vi "KepcoDCPwr Query Voltage Limit.vi"(0 "VISA Session":refnum<visa-resource-name>, 5 "Model In":string, 7 "channel name (\"\")":string="\"\"", 9 "Max Level (T),MIN LEVEL(F)":bool caption="Level", 11 "error in (no error)":errorcluster {"code" format="%.0x"}) -> (4 "VISA Session Out":refnum<visa-resource-name>, 6 "Model Out":string, 8 "channel name out (\"\")":string="\"\"" caption="channel name Out (\"\")", 10 "voltage level":dbl format="%^.2e", 15 "error out":errorcluster {"code" format="%.0x"})   [LabVIEW 2013]
doc: "This VI returns the maximum programmable voltage level that the power supply accepts for a particular current limit on a channel for the output range to which the power supply is currently configured."
uses:
  <vilib>/regexp/Match Regular Expression.xnode
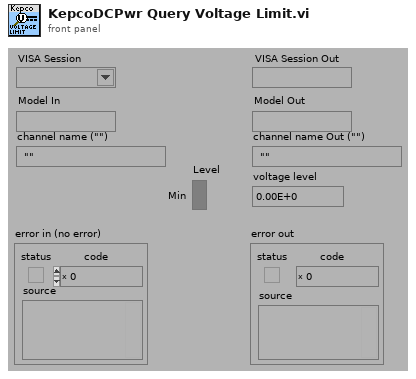
[diagram p1: front panel]
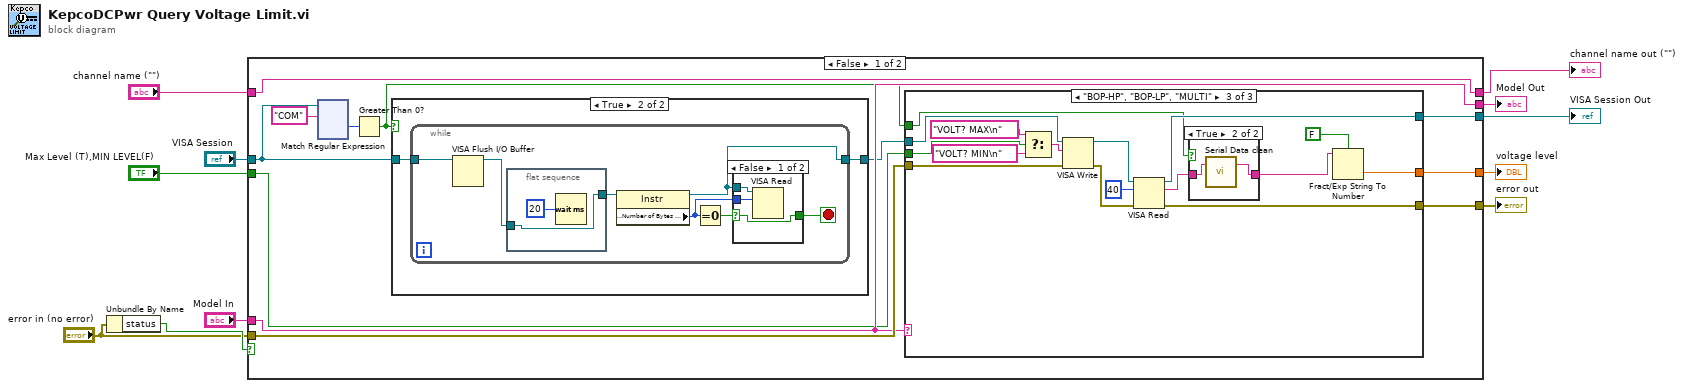
[diagram p0: block diagram]
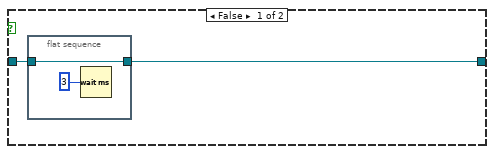
[diagram p2: hidden frame]
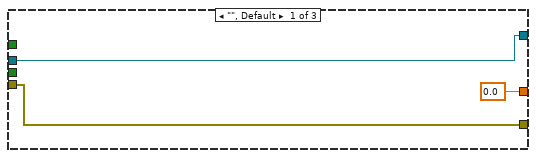
[diagram p4: hidden frame]
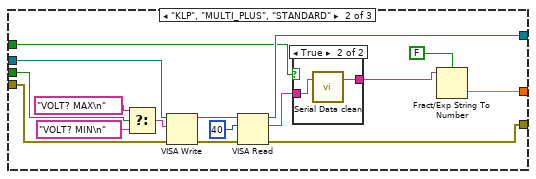
[diagram p5: hidden frame]
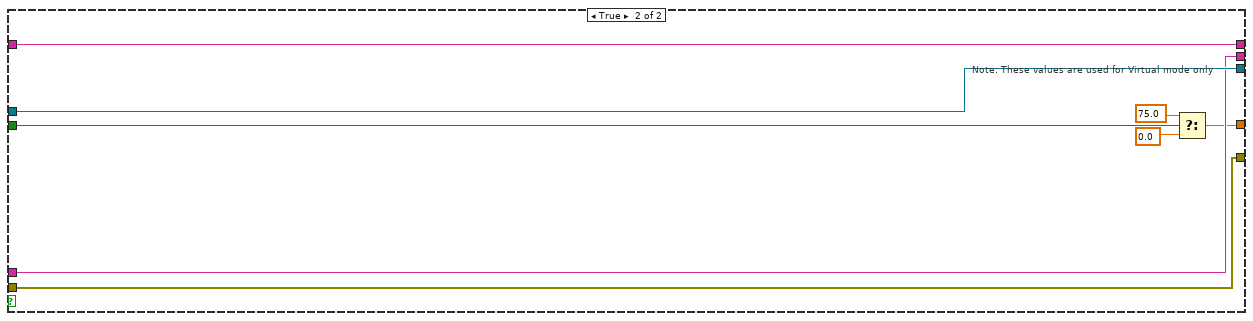
[diagram p8: hidden frame]
diagram:
  n1 = Unbundle By Name("error in (no error)") -> ("status"=w10:bool)
  n2 = case shown="False" w10 {
    tunnel: [w19 w202] -> w11
    tunnel: "error in (no error)" -> [w22 w202]
    tunnel: [w20 w201] -> w5
    tunnel: "VISA Session" -> [w12 w201]
    tunnel: [w21 w200] -> w4
    tunnel: "Model In" -> [w21 w200]
    tunnel: [w23 w199] -> w3
    tunnel: "channel name (\"\")" -> [w23 w199]
    tunnel: [w18 w196] -> w2
    tunnel: "Max Level (T),MIN LEVEL(F)" -> [w17 w198]
    frame False {
      n3 = xnode "Match Regular Expression"("input string"=w12, "regular expression"="COM") -> ("offset past match"=w15:i32)  [unwired: 2 in, 6 out]
      n4 = Greater Than 0?(x=w15) -> (x > 0?=w14:bool)
      n5 = case shown="True" w14 {
        tunnel: [w25 w29] -> w13
        tunnel: w12 -> [w24 w28]
        frame False {
          n6 = flat-sequence {
            tunnel: w24 -> [w27]
            tunnel: [w27] -> w25
            frame #0 {
              n7 = Wait (ms)(milliseconds to wait=u32 3 ("byte count (0)")) -> ()  [unwired: 1 out]
            }
          }
        }
        frame True {
          n8 = while {
            tunnel: w28 -> [w32]
            tunnel: [w34] -> w29
            stop <- w35 stop-if-true
            n9 = VISA Flush I/O Buffer(VISA resource name=w32) -> (VISA resource name out=w31:refnum<visa-resource-name>)  [unwired: 2 in, 1 out]
            n10 = flat-sequence {
              tunnel: w31 -> [w37]
              tunnel: [w37] -> w30
              frame #0 {
                n11 = Wait (ms)(milliseconds to wait=u32 20) -> ()  [unwired: 1 out]
              }
            }
            n12 = property class="Instr"(reference=w30) -> (reference out=w34:refnum<visa-resource-name>, "Serial Settings:Number of Bytes at Serial Port"=w33:u32)  [unwired: 1 in, 1 out]
            n13 = Equal To 0?(x=w33) -> (x = 0?=w36:bool)
            n14 = case shown="False" w36 {
              selector: w36 -> [w41 w42]
              tunnel: [w41 w42] -> w35
              tunnel: w34 -> [w40 _]
              tunnel: w33 -> [w39 _]
              frame False {
                n15 = VISA Read(VISA resource name=w40, byte count=w39) -> ()  [unwired: 1 in, 4 out]
              }
              frame True {
              }
            }
          }
        }
      }
      n16 = case shown="\"BOP-HP\", \"BOP-LP\", \"MULTI\"" w21 {
        tunnel: w22 -> [w154 w172 w191]
        tunnel: w13 -> [w155 w171 w176]
        tunnel: [w155 w169 w190] -> w20
        tunnel: [w154 w168 w189] -> w19
        tunnel: [0.0 w166 w188] -> w18
        tunnel: w17 -> [_ w164 w186]
        tunnel: w14 -> [_ w159 w181]
        frame "", Default {
        }
        frame "KLP", "MULTI_PLUS", "STANDARD" {
          n17 = Select(t="VOLT? MAX\n", s=w164, f="VOLT? MIN\n") -> (s? t:f=w161:string)
          n18 = VISA Write(VISA resource name=w171, write buffer=w161, error in (no error)=w172) -> (VISA resource name out=w170:refnum<visa-resource-name>, error out=w167:errorcluster)  [unwired: 1 out]
          n19 = VISA Read(VISA resource name=w170, byte count=u32 40 ("byte count (0)"), error in (no error)=w167) -> (VISA resource name out=w169:refnum<visa-resource-name>, read buffer=w157:string, error out=w168:errorcluster)  [unwired: 1 out]
          n20 = case shown="True" w159 {
            tunnel: [w173 w174] -> w158
            tunnel: w157 -> [w173 w175]
            frame False {
            }
            frame True {
              n21 = call "Serial Data clean.vi"("string"=w175) -> ("Stripped of Xon Xoff"=w174:string)  [unwired: 2 in]
            }
          }
          n22 = Fract/Exp String To Number(use system decimal point (T)=FALSE, string=w158) -> (number=w166:dbl)  [unwired: 2 in, 1 out]
        }
        frame "BOP-HP", "BOP-LP", "MULTI" {
          n23 = Select(t="VOLT? MAX\n", s=w186, f="VOLT? MIN\n") -> (s? t:f=w183:string)
          n24 = VISA Write(VISA resource name=w176, write buffer=w183, error in (no error)=w191) -> (VISA resource name out=w180:refnum<visa-resource-name>, error out=w179:errorcluster)  [unwired: 1 out]
          n25 = VISA Read(VISA resource name=w180, byte count=u32 40 ("byte count (0)"), error in (no error)=w179) -> (VISA resource name out=w190:refnum<visa-resource-name>, read buffer=w178:string, error out=w189:errorcluster)  [unwired: 1 out]
          n26 = case shown="True" w181 {
            tunnel: w178 -> [w192 w193]
            tunnel: [w192 w194] -> w177
            frame False {
            }
            frame True {
              n27 = call "Serial Data clean.vi"("string"=w193) -> ("Stripped of Xon Xoff"=w194:string)  [unwired: 2 in]
            }
          }
          n28 = Fract/Exp String To Number(use system decimal point (T)=FALSE, string=w177) -> (number=w188:dbl)  [unwired: 2 in, 1 out]
        }
      }
    }
    frame True {
      # "Note: These values are used for Virtual mode only"
      n29 = Select(t=75.0, s=w198, f=0.0) -> (s? t:f=w196:dbl)
    }
  }
  "error out" <- w11
  "channel name out (\"\")" <- w3
  "Model Out" <- w4
  "VISA Session Out" <- w5
  "voltage level" <- w2
